vi "NameMapping_read.vi"(8 "error in (no error)":errorcluster) -> (0 "error out":errorcluster, 1 "AE-Names Mapping":T1(array[cluster]), 2 "AE-Names (Filter)":cluster{"String":string, "String":string}[](array[cluster]), 3 "AE-List":string[](array[string]))   [LabVIEW 2017, in "MainFrameLib.lvlib"]
uses:
  MainFrameLib.lvlib
  <vilib>/Utility/file.llb/Read Delimited Spreadsheet (string).vi
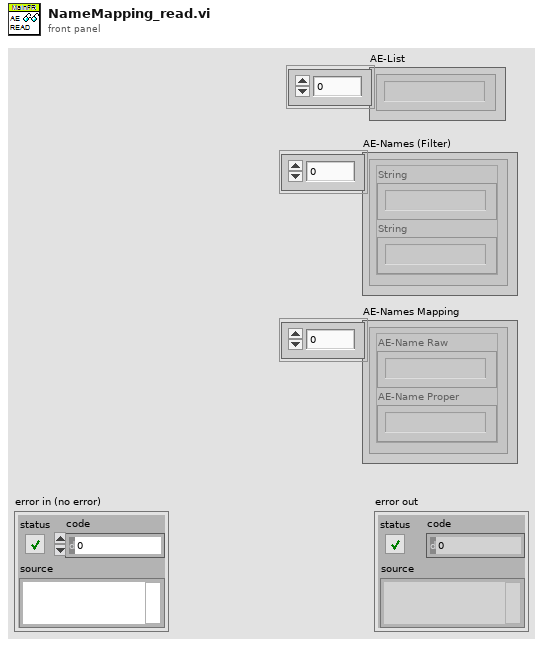
[diagram p1: front panel]
types:
  T1 = cluster{"AE-Name Raw":string, "AE-Name Proper":string}[]
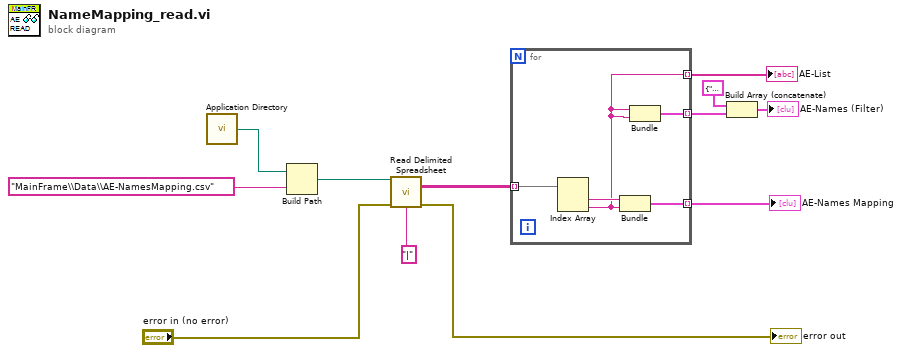
[diagram p0: block diagram]
diagram:
  n1 = call <vilib>:"Application Directory.vi"() -> ("Application Directory"=w12:path)
  n2 = Build Path(base path=w12, name or relative path="MainFrame\\Data\\AE-NamesMapping.csv") -> (appended path=w10:path)
  n3 = call-poly <vilib>:"Read Delimited Spreadsheet.vi"("file path (dialog if empty)"=w10, "error in (no error)"="error in (no error)", "delimiter (\\t)"="|" ("delimiter (\\t)")) -> ("all rows"=w8:string[][], "error out"=→"error out":errorcluster)  [unwired: 7 in, 4 out]
  n4 = for {
    tunnel: w8 -> [w17] mode=indexing
    tunnel: [w15] -> w7 mode=indexing
    tunnel: [w14] -> w3 mode=indexing
    tunnel: [w13] -> w4 mode=indexing
    n5 = Index Array(array=w17) -> (element #1=w16:string, element #2=w13:string)  [unwired: 2 in]
    n6 = Bundle("String"=w16, "String"=w13) -> (w15:cluster{"String":string, "String":string})  [unwired: 1 in]
    n7 = Bundle("String"=w13, "String"=w13) -> (w14:cluster{"String":string, "String":string})  [unwired: 1 in]
  }
  "AE-Names Mapping" <- w7
  "AE-List" <- w4
  n8 = Build Array (concatenate)(cluster{"String":string, "String":string} {"String"="Default", "String"="AE Selection"} ("output cluster"), w3) -> (→"AE-Names (Filter)":cluster{"String":string, "String":string}[])
